vi "ziSetValueBinary.vi"(3 "Error In":errorcluster, 4 "Data":string, 5 "Path":string, 6 "Handle In":T1 {"Handle" format="0x%08x"; "Conn" format="0x%08x"}) -> (0 "Error Out":errorcluster, 2 "Handle Out":T1 {"Handle" format="0x%08x"; "Conn" format="0x%08x"})   [LabVIEW 2015, in "Zurich Instruments LabOne.lvlib"]
doc: "This vi writes the string as bytes of binary data to the nodes specified by <b>Path</b>. More than one node can be set if a wildcard is used in <b>Path</b>."
uses:
  Zurich Instruments LabOne.lvlib
  Zurich Instruments/LabOne/API/LabVIEW/Zurich Instruments LabOne/Private/ziLV64.framework
  ziTypeHandle.ctl
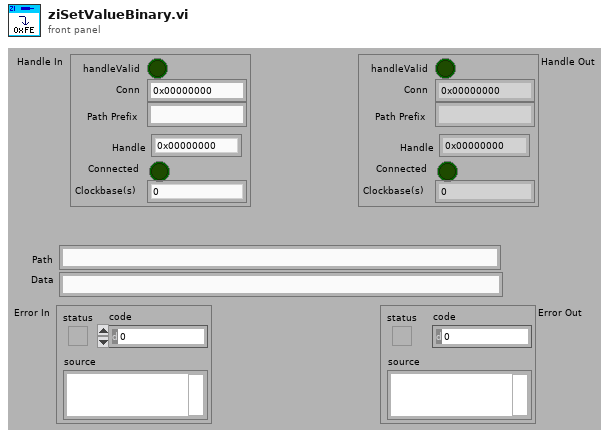
[diagram p1: front panel]
types:
  T1 = typedef "Zurich Instruments LabOne.lvlib/ziTypeHandle.ctl" = cluster{"handleValid":bool, "Conn":u64, "Path Prefix":string, "Handle":u64, "Connected":bool, "Clockbase(s)":dbl}
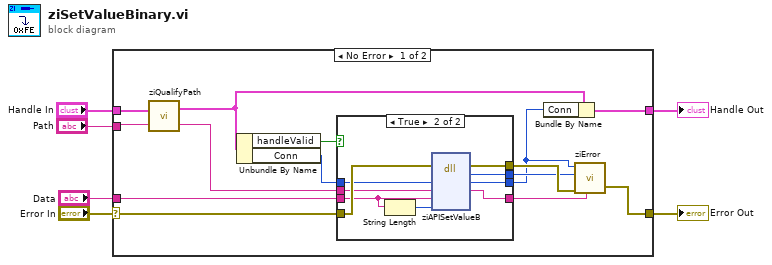
[diagram p0: block diagram]
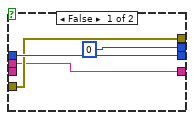
[diagram p2: hidden frame]
diagram:
  n1 = case shown="No Error" "Error In" {
    selector: "Error In" -> [w8 w35]
    tunnel: "Data" -> [w19 _]
    tunnel: [w18 w35] -> w5
    tunnel: [w14 w34] -> w4
    tunnel: "Handle In" -> [w13 w34]
    tunnel: "Path" -> [w11 _]
    frame No Error {
      n2 = call "ziQualifyPath.vi"("Path In"=w11, "Handle In"=w13) -> ("Path Out"=w10:string, "Handle Out"=w12:T1)
      n3 = Unbundle By Name(w12) -> ("handleValid"=w15:bool, "Conn"=w20:u64)
      n4 = case shown="True" w15 {
        tunnel: w8 -> [w23 w33]
        tunnel: w20 -> [w24 w32]
        tunnel: w10 -> [w21 w31]
        tunnel: w19 -> [_ w26]
        tunnel: [w23 w30] -> w17
        tunnel: [u32 0 ("return type") w29] -> w16
        tunnel: [w24 w28] -> w7
        tunnel: [w21 w27] -> w9
        frame False {
        }
        frame True {
          n5 = String Length(string=w26) -> (length=w25:i32)
          n6 = dll-call lib="Users/arkady/Desktop/ado/github/resonant_ultrasound_arxiv/maglab ultrasound -- arkady --arxiv/Zurich Instruments/LabOne/API/LabVIEW/Zurich Instruments LabOne/Private/ziLV*.*" fn="ziAPISetValueB"(error in=w33, "Conn"=w32, "Path"=w31, "Value"=w26, "Len"=w25) -> (error out=w30:errorcluster, "return type"=w29:u32, "Conn"=w28:u64, "Path"=w27:string)  [unwired: 4 in, 1 out]
        }
      }
      n7 = Bundle By Name(cluster=w12, "Conn"=w7) -> (w14:T1)
      n8 = call "ziError.vi"("Conn"=w7, "ziErrorCode"=w16, "Error In"=w17, "Annotation"=w9) -> ("Error Out"=w18:errorcluster)  [unwired: 1 in, 1 out]
    }
    frame Error {
    }
  }
  "Error Out" <- w5
  "Handle Out" <- w4
